vi "Pickering action.vi"(4 "Initialize":bool, 5 "Pickering status":path=path "C:/LabView/PPMS basic VIs/Switch Status.txt", 6 "Action":enum16{"Close", "Open", "Disconnect all"}(ring), 7 "option string":string="Simulate=0,RangeCheck=1,QueryInstrStatus=0,Cache=1,DriverSetup=Model:40-726-511-M;", 8 "error in (no error)":errorcluster, 10 "Channels Array":T2=[{"Channel x"="x12", "Channel y"="y1"}, {"Channel x"="x12", "Channel y"="y2"}, {"Channel x"="x12", "Channel y"="y3"}, {"Channel x"="x12", "Channel y"="y4"}, {"Channel x"="x12", "Channel y"="y5"}, {"Channel x"="x12", "Channel y"="y6"}, {"Channel x"="x12", "Channel y"="y7"}, {"Channel x"="x12", "Channel y"="y8"}], 11 "instrument handle":string="PXI9::13::INSTR") -> (0 "error out":errorcluster, 3 "instrument handle out":string="PXI9::13::INSTR (2)")   [LabVIEW 2016, in "pickering.lvclass"]
uses:
  pickering.lvclass
  Typedefs/Channels-Array.ctl
  Typedefs/Channel-Cluster.ctl
  Typedefs/ChannelX-ComboBox.ctl
  Typedefs/ChannelY-ComboBox.ctl
panel:
  out "Additionally Connected Switches":T1(array[cluster])=[{"result string"="xA5", "result string"="yA7"}, {"result string"="comC5", "result string"="chC5"}, {"result string"="comD7", "result string"="chD7"}, {"result string"="xA8", "result string"="yA4"}, {"result string"="xA8", "result string"="yA8"}, {"result string"="comC8", "result string"="chC8"}, {"result string"="xA1", "result string"="yA3"}, {"result string"="comD3", "result string"="chD3"}, {"result string"="xA3", "result string"="yA5"}, {"result string"="comC3", "result string"="chC3"}, {"result string"="comD5", "result string"="chD5"}]
  out "Disconnected Switches":T1(array[cluster])=[{"result string"="xA12", "result string"="yA1"}, {"result string"="comB12", "result string"="chB12"}, {"result string"="xA12", "result string"="yA2"}, {"result string"="comE2", "result string"="chE2"}, {"result string"="xA12", "result string"="yA3"}, {"result string"="comE3", "result string"="chE3"}, {"result string"="xA12", "result string"="yA4"}, {"result string"="xA12", "result string"="yA5"}, {"result string"="comC12", "result string"="chC12"}, {"result string"="comE5", "result string"="chE5"}, {"result string"="xA12", "result string"="yA6"}, {"result string"="comE6", "result string"="chE6"}, {"result string"="xA12", "result string"="yA7"}, {"result string"="comE7", "result string"="chE7"}, {"result string"="xA12", "result string"="yA8"}, {"result string"="xA1", "result string"="yA1"}, {"result string"="comD1", "result string"="chD1"}, {"result string"="xA2", "result string"="yA1"}, {"result string"="comB2", "result string"="chB2"}, {"result string"="xA3", "result string"="yA1"}, {"result string"="comB3", "result string"="chB3"}, {"result string"="xA4", "result string"="yA1"}, {"result string"="comB4", "result string"="chB4"}, {"result string"="xA5", "result string"="yA1"}, {"result string"="comB5", "result string"="chB5"}, {"result string"="xA6", "result string"="yA1"}, {"result string"="comB6", "result string"="chB6"}, {"result string"="xA8", "result string"="yA1"}, {"result string"="xA9", "result string"="yA1"}, {"result string"="comB9", "result string"="chB9"}, {"result string"="xA10", "result string"="yA1"}, {"result string"="comB10", "result string"="chB10"}, {"result string"="xA11", "result string"="yA1"}, {"result string"="comB11", "result string"="chB11"}]
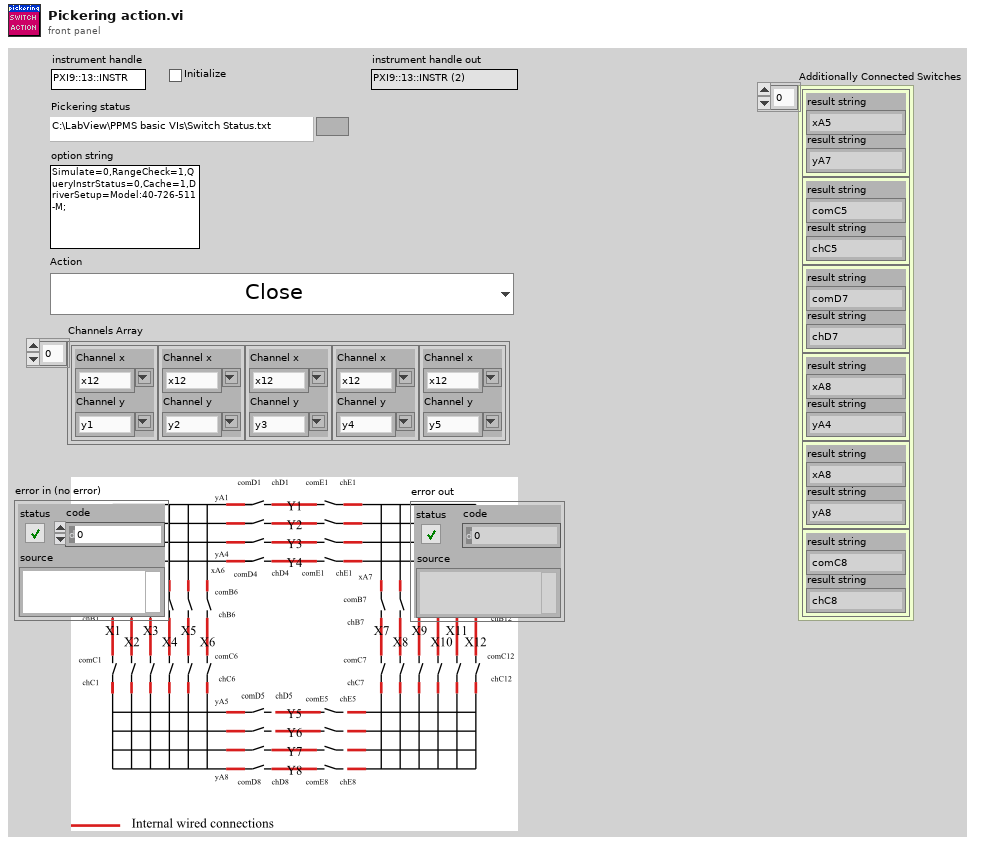
[diagram p1: front panel]
types:
  T1 = cluster{"result string":string, "result string":string}[]
  T2 = typedef "pickering.lvclass/Channels-Array.ctl" = T3[]
  T3 = typedef "pickering.lvclass/Channel-Cluster.ctl" = cluster{"Channel x":T4, "Channel y":T5}
  T4 = typedef "pickering.lvclass/ChannelX-ComboBox.ctl" = string
  T5 = typedef "pickering.lvclass/ChannelY-ComboBox.ctl" = string
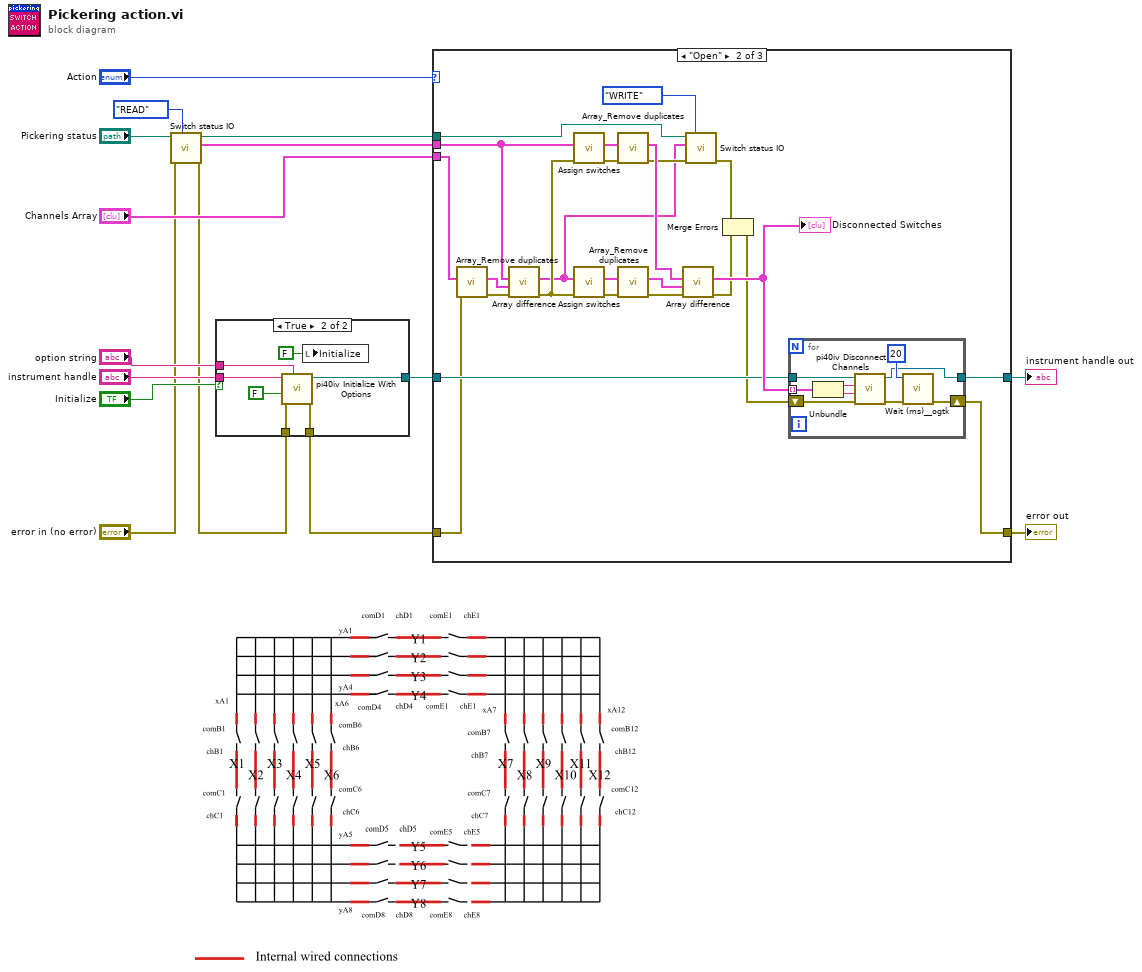
[diagram p0: block diagram]
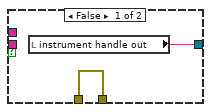
[diagram p2: hidden frame]
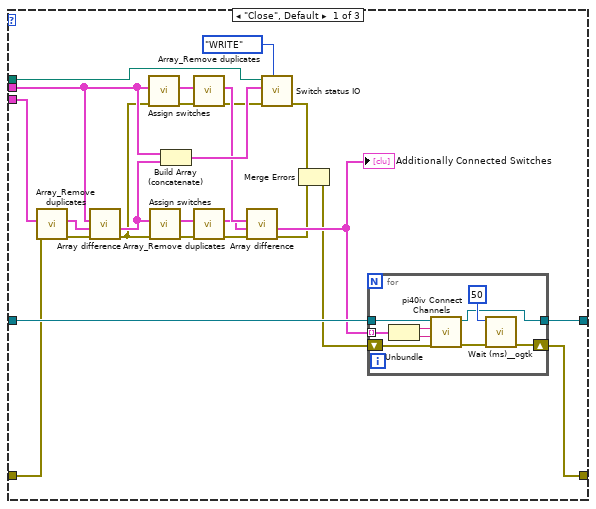
[diagram p3: hidden frame]
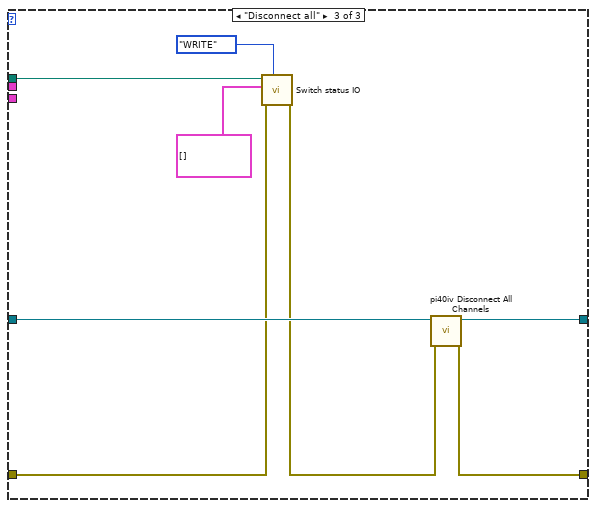
[diagram p4: hidden frame]
diagram:
  n1 = call "Switch status IO.vi"("mode"=enum16{"READ", "WRITE"}."READ", "error in (no error)"="error in (no error)", "Path"="Pickering status") -> ("error out"=w4:errorcluster, "Channels out"=w8:T2, "Path out"=w7:path)  [unwired: 6 in]
  n2 = case shown="True" "Initialize" {
    tunnel: "instrument handle" -> [_ w24]
    tunnel: "option string" -> [_ w22]
    tunnel: [w17 w23] -> w10
    tunnel: w4 -> [w16 w19]
    tunnel: [w16 w18] -> w1
    frame False {
      n3 = local read "instrument handle out"() -> (w17:string)
    }
    frame True {
      n4 = call <instrlib>:"pi40iv Initialize With Options.vi"("option string"=w22, "error in (no error)"=w19, "reset device"=FALSE, "resource name"=w24) -> ("error out"=w18:errorcluster, "instrument handle out"=w23:refnum<k15>)  [unwired: 6 in]
      n5 = local write "Initialize"(FALSE ("Initialize")) -> ()
    }
  }
  n6 = case shown="\"Open\"" "Action" {
    tunnel: w10 -> [w49 w80 w99]
    tunnel: "Channels Array" -> [w40 w77 _]
    tunnel: w7 -> [w32 w68 w98]
    tunnel: w8 -> [w38 w71 _]
    tunnel: [w41 w75 w96] -> w9
    tunnel: w1 -> [w26 w65 w92]
    tunnel: [w28 w64 w93] -> w2
    frame "Close", Default {
      n7 = call "Array_Remove duplicates.vi"("error in (no error)"=w26, "Array Input"=w40) -> ("error out"=w37:errorcluster, "Array Output"=w39:T2)  [unwired: 8 in]
      n8 = call "Array difference.vi"("error in (no error)"=w37, "Channels Array 2"=w39, "Channels Array"=w38) -> ("error out"=w31:errorcluster, "Array 2-(array1&2)"=w47:T2)  [unwired: 6 in, 1 out]
      n9 = call "Assign switches.vi"("error in (no error)"=w31, "Channel Array In"=w38) -> ("error out"=w34:errorcluster, "Channel Array Out"=w45:T2)  [unwired: 8 in]
      n10 = call "Assign switches.vi"("error in (no error)"=w31, "Channel Array In"=w47) -> ("error out"=w36:errorcluster, "Channel Array Out"=w46:T2)  [unwired: 8 in]
      n11 = Build Array (concatenate)(w38, w47) -> (w48:T2)
      n12 = call "Array_Remove duplicates.vi"("error in (no error)"=w34, "Array Input"=w45) -> ("error out"=w27:errorcluster, "Array Output"=w44:T2)  [unwired: 8 in]
      n13 = call "Array_Remove duplicates.vi"("error in (no error)"=w36, "Array Input"=w46) -> ("error out"=w35:errorcluster, "Array Output"=w43:T2)  [unwired: 8 in]
      n14 = call "Array difference.vi"("error in (no error)"=w35, "Channels Array 2"=w43, "Channels Array"=w44) -> ("error out"=w30:errorcluster, "Array 2-(array1&2)"=w42:T2)  [unwired: 6 in, 1 out]
      "Additionally Connected Switches" <- w42
      n15 = call "Switch status IO.vi"("mode"=enum16{"READ", "WRITE"}."WRITE", "error in (no error)"=w27, "Channels in"=w48, "Path"=w32) -> ("error out"=w25:errorcluster)  [unwired: 5 in, 2 out]
      n16 = Merge Errors(w25, w30) -> (w29:errorcluster)
      n17 = for {
        tunnel: w49 -> [w58]
        tunnel: w42 -> [w57] mode=indexing
        tunnel: [w50] -> w41
        shift-right: [w51] -> w28
        shift-left: w29 -> [w52]
        n18 = Unbundle(w57) -> ("Channel x"=w56:T4, "Channel y"=w55:T5)
        n19 = call <instrlib>:"pi40iv Connect Channels.vi"("error in (no error)"=w52, "channel 2"=w55, "channel 1"=w56, "instrument handle"=w58) -> ("error out"=w53:errorcluster, "instrument handle out"=w50:refnum<k15>)  [unwired: 6 in]
        n20 = call <userlib>:"Wait (ms)__ogtk.vi"("error in (no error)"=w53, "milliseconds to wait"=u32 50) -> ("error out"=w51:errorcluster)  [unwired: 8 in, 1 out]
      }
    }
    frame "Open" {
      n21 = call "Array_Remove duplicates.vi"("error in (no error)"=w65, "Array Input"=w77) -> ("error out"=w72:errorcluster, "Array Output"=w76:T2)  [unwired: 8 in]
      n22 = call "Array difference.vi"("error in (no error)"=w72, "Channels Array 2"=w76, "Channels Array"=w71) -> ("error out"=w66:errorcluster, "Array 1-(array1&2)"=w59:T2)  [unwired: 6 in, 1 out]
      n23 = call "Assign switches.vi"("error in (no error)"=w66, "Channel Array In"=w71) -> ("error out"=w70:errorcluster, "Channel Array Out"=w79:T2)  [unwired: 8 in]
      n24 = call "Assign switches.vi"("error in (no error)"=w66, "Channel Array In"=w59) -> ("error out"=w74:errorcluster, "Channel Array Out"=w78:T2)  [unwired: 8 in]
      n25 = call "Array_Remove duplicates.vi"("error in (no error)"=w70, "Array Input"=w79) -> ("error out"=w60:errorcluster, "Array Output"=w67:T2)  [unwired: 8 in]
      n26 = call "Array_Remove duplicates.vi"("error in (no error)"=w74, "Array Input"=w78) -> ("error out"=w73:errorcluster, "Array Output"=w82:T2)  [unwired: 8 in]
      n27 = call "Array difference.vi"("error in (no error)"=w73, "Channels Array 2"=w82, "Channels Array"=w67) -> ("error out"=w62:errorcluster, "Array 1-(array1&2)"=w81:T2)  [unwired: 6 in, 1 out]
      "Disconnected Switches" <- w81
      n28 = call "Switch status IO.vi"("mode"=enum16{"READ", "WRITE"}."WRITE", "error in (no error)"=w60, "Channels in"=w59, "Path"=w68) -> ("error out"=w63:errorcluster)  [unwired: 5 in, 2 out]
      n29 = Merge Errors(w63, w62) -> (w61:errorcluster)
      n30 = for {
        tunnel: w81 -> [w91] mode=indexing
        tunnel: w80 -> [w88]
        tunnel: [w85] -> w75
        shift-right: [w84] -> w64
        shift-left: w61 -> [w83]
        n31 = Unbundle(w91) -> ("Channel x"=w90:T4, "Channel y"=w89:T5)
        n32 = call <instrlib>:"pi40iv Disconnect Channels.vi"("error in (no error)"=w83, "channel 2"=w89, "channel 1"=w90, "instrument handle"=w88) -> ("error out"=w87:errorcluster, "instrument handle out"=w85:refnum<k15>)  [unwired: 6 in]
        n33 = call <userlib>:"Wait (ms)__ogtk.vi"("error in (no error)"=w87, "milliseconds to wait"=u32 20) -> ("error out"=w84:errorcluster)  [unwired: 8 in, 1 out]
      }
    }
    frame "Disconnect all" {
      n34 = call "Switch status IO.vi"("mode"=enum16{"READ", "WRITE"}."WRITE", "error in (no error)"=w92, "Channels in"=T2 [] ("String input"), "Path"=w98) -> ("error out"=w94:errorcluster)  [unwired: 5 in, 2 out]
      n35 = call <instrlib>:"pi40iv Disconnect All Channels.vi"("error in (no error)"=w94, "instrument handle"=w99) -> ("error out"=w93:errorcluster, "instrument handle out"=w96:refnum<k15>)  [unwired: 8 in]
    }
  }
  "instrument handle out" <- w9
  "error out" <- w2
